vi "Load Profile.vi"(0 "Output":bool, 7 "output cluster":T1) -> (4 "error out":errorcluster)   [LabVIEW 2017]
uses:
  <vilib>/Utility/file.llb/Read Delimited Spreadsheet (DBL).vi
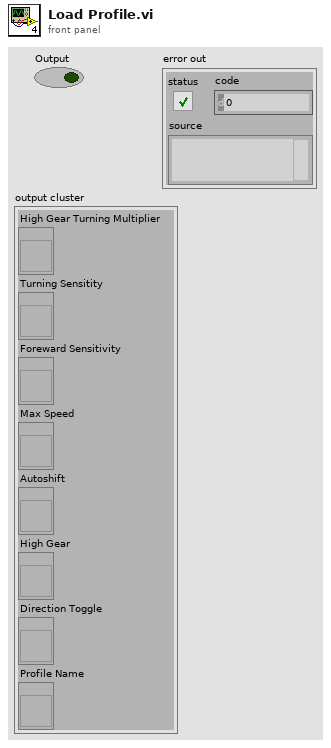
[diagram p1: front panel]
types:
  T1 = cluster{"High Gear Turning Multiplier":refnum<vi>, "Turning Sensitity":refnum<vi>, "Foreward Sensitivity":refnum<vi>, "Max Speed":refnum<vi>, "Autoshift":refnum<vi>, "High Gear":refnum<vi>, "Direction Toggle":refnum<vi>, "Profile Name":refnum<vi>}
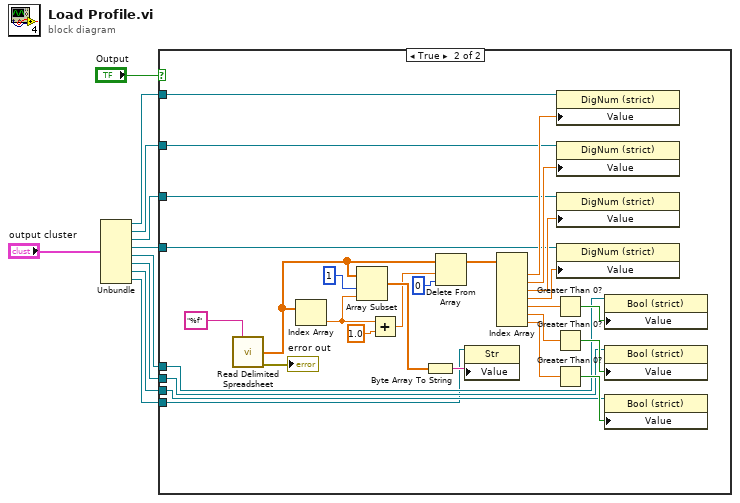
[diagram p0: block diagram]
diagram:
  n1 = Unbundle("output cluster") -> ("High Gear Turning Multiplier"=w8:refnum<vi>, "Turning Sensitity"=w7:refnum<vi>, "Foreward Sensitivity"=w6:refnum<vi>, "Max Speed"=w5:refnum<vi>, "Autoshift"=w4:refnum<vi>, "High Gear"=w3:refnum<vi>, "Direction Toggle"=w2:refnum<vi>, "Profile Name"=w1:refnum<vi>)
  n2 = case shown="True" "Output" {
    tunnel: w4 -> [_ w18]
    tunnel: w3 -> [_ w17]
    tunnel: w2 -> [_ w16]
    tunnel: w5 -> [_ w15]
    tunnel: w6 -> [_ w14]
    tunnel: w7 -> [_ w13]
    tunnel: w8 -> [_ w12]
    tunnel: w1 -> [_ w11]
    frame False {
    }
    frame True {
      n3 = call-poly <vilib>:"Read Delimited Spreadsheet.vi"("format (%.3f)"="%f") -> ("first row"=w36:dbl[], "error out"=→"error out":errorcluster)  [unwired: 9 in, 4 out]
      n4 = Index Array(array=w36) -> (element=w19:dbl)  [unwired: 1 in]
      n5 = Array Subset(array=w36, index=1, length=w19) -> (w37:dbl[])
      n6 = Add(x=w19, y=1.0) -> (x+y=w21:dbl)
      n7 = Byte Array To String(unsigned byte array=w37) -> (string=w23:string)
      n8 = Delete From Array(array=w36, length=w21, index=0) -> (array with subset deleted=w34:dbl[])  [unwired: 1 out]
      n9 = property on="Property Node" class="Str"(reference=w11, "Value"=w23) -> ()  [unwired: 1 in, 2 out]
      n10 = Index Array(array=w34) -> (element #1=w33:dbl, element #2=w32:dbl, element #3=w31:dbl, element #4=w30:dbl, element #5=w29:dbl, element #6=w28:dbl, element #7=w27:dbl)  [unwired: 7 in]
      n11 = Greater Than 0?(x=w29) -> (x > 0?=w24:bool)
      n12 = Greater Than 0?(x=w28) -> (x > 0?=w25:bool)
      n13 = Greater Than 0?(x=w27) -> (x > 0?=w26:bool)
      n14 = property on="Property Node" class="DigNum (strict)"(reference=w12, "Value"=w33) -> ()  [unwired: 1 in, 2 out]
      n15 = property on="Property Node" class="DigNum (strict)"(reference=w13, "Value"=w32) -> ()  [unwired: 1 in, 2 out]
      n16 = property on="Property Node" class="DigNum (strict)"(reference=w14, "Value"=w31) -> ()  [unwired: 1 in, 2 out]
      n17 = property on="Property Node" class="DigNum (strict)"(reference=w15, "Value"=w30) -> ()  [unwired: 1 in, 2 out]
      n18 = property on="Property Node" class="Bool (strict)"(reference=w18, "Value"=w24) -> ()  [unwired: 1 in, 2 out]
      n19 = property on="Property Node" class="Bool (strict)"(reference=w17, "Value"=w25) -> ()  [unwired: 1 in, 2 out]
      n20 = property on="Property Node" class="Bool (strict)"(reference=w16, "Value"=w26) -> ()  [unwired: 1 in, 2 out]
    }
  }
